vi "TX_单音扫频.vi"() -> ()   [LabVIEW 2015]
uses:
  <vilib>/Instr/_visa.llb/VISA Configure Serial Port (Instr).vi
  <instrlib>/Agilent E363X Series/Agilent E363X Series.lvlib
  <instrlib>/Rohde&Schwarz Spectrum Analyzer/Rohde&Schwarz Spectrum Analyzer.lvlib
panel:
  in  "type specifier VI Refnum (for type only)":refnum<vi>
  in  "Stop Frequency (0.0) 2":dbl=2130000000.0 caption="Stop Frequency (0.0)" format="%#.9p"
  in  "Start Frequency (0.0) 2":dbl=2000000000.0 caption="Start Frequency (0.0)" format="%#.9p"
  in  "Stop Frequency (0.0)":dbl=2130000000.0 format="%#.9p"
  in  "Start Frequency (0.0)":dbl=2000000000.0 format="%#.9p"
  in  "模板路径 2":path=path "E:/Everst_TestReport/Everst_TestReport_Template.xlsx"
  in  "测试板编号 2":i32=4
  in  "保存路径 2":path=path "E:/Everst_TestReport/Report/Everrst_#"
  in  "开关":bool[](array[boolean])=[FALSE, TRUE, TRUE, FALSE, FALSE, FALSE, FALSE, TRUE, TRUE, FALSE]
  out "volt2v":dbl[](array[numeric])
  out "volt1v3":dbl[](array[numeric])
  in  "error in (no error) 6":errorcluster {"code" format="%.0x"}
  in  "error in (no error) 5":errorcluster caption="error in (no error)"
  in  "error in (no error) 4":errorcluster caption="error in (no error)"
  in  "error in (no error) 3":errorcluster
  in  "error in (no error) 2":errorcluster
  in  "error in (no error)":errorcluster
  in  "直流电源2v":refnum<visa-resource-name>="GPIB0::6::INSTR"
  in  "Frequency (1.0e9 Hz)":dbl=10000000.0 format="%.3f"
  in  "RF Output Level (-30.0 dBm)":dbl=10.0 caption="RF Output Level (-30.0)" format="%.3f"
  in  "Reference Level Offset (0.0) 2":dbl=0.95 caption="Reference Level Offset (0.0)" format="%^.3e"
  in  "Coupling Value (0.0) 2":dbl=200000.0 caption="Coupling Value (0.0)" format="%^.3e"
  in  "Reference Level (-20.0) 2":dbl=30.0 caption="Reference Level (-20.0)" format="%^.3e"
  in  "Span (0.0) 2":dbl=1000000000.0 caption="Span (0.0)" format="%.1f"
  in  "Center Frequency (0.0) 2":dbl=2100000000.0 caption="Center Frequency (0.0)" format="%#.9p"
  in  "Reference Level Offset (0.0)":dbl=2.3 format="%^.3e"
  in  "Coupling Value (0.0)":dbl=200000.0 format="%^.3e"
  in  "Reference Level (-20.0)":dbl=30.0 format="%^.3e"
  in  "Span (0.0)":dbl=1000000000.0 format="%.1f"
  in  "Center Frequency (0.0)":dbl=2100000000.0 format="%#.9p"
  in  "配置文件路径":path=path "E:/Everst_TestReport/config.xlsx"
  out "Bamp_next":dbl[](array[numeric])
  out "Bamp_max":dbl[](array[numeric])
  in  "Marker Search 4":i32(ring)=1 caption="Marker Search" items=["Peak Maximum"=1, "Peak Minimum"=2, "Next Maximum"=3, "Left Maximum"=4, "Right Maximum"=5, "Next Minimum"=6, "Left Minimum"=7, "Right Minimum"=8]
  in  "Peak Excursion 4":dbl=3.0 caption="Peak Excursion" format="%.1f"
  out "channelB_y1":dbl[](array[numeric]) caption="Amplitude" format="%^.3e"
  out "channelB_x1":dbl[](array[numeric]) caption="X" format="%^.3e"
  out "Apos_next":dbl[](array[numeric])
  in  "Aamp_next":dbl[](array[numeric])
  out "Aamp_max":dbl[](array[numeric])
  out "Apos_max":dbl[](array[numeric])
  in  "Marker Search 3":i32(ring)=1 caption="Marker Search" items=["Peak Maximum"=1, "Peak Minimum"=2, "Next Maximum"=3, "Left Maximum"=4, "Right Maximum"=5, "Next Minimum"=6, "Left Minimum"=7, "Right Minimum"=8]
  in  "Peak Excursion 3":dbl=3.0 caption="Peak Excursion" format="%.1f"
  out "channelA_y1":dbl[](array[numeric]) caption="Amplitude" format="%^.3e"
  out "channelA_x1":dbl[](array[numeric]) caption="X" format="%^.3e"
  out "fin_dac":dbl[](array[numeric])
  in  "信号发生器地址":refnum<visa-resource-name>="GPIB0::10::INSTR"
  in  "频谱仪地址B":refnum<visa-resource-name>="TCPIP0::192.168.1.4::inst0::INSTR"
  in  "频谱仪地址A":refnum<visa-resource-name>="GPIB0::22::INSTR"
  in  "直流电源(1.3V)":refnum<visa-resource-name>="GPIB0::4::INSTR"
  in  "FPGA串口地址":refnum<visa-resource-name>="COM3"
  out "fin":dbl[](array[numeric])
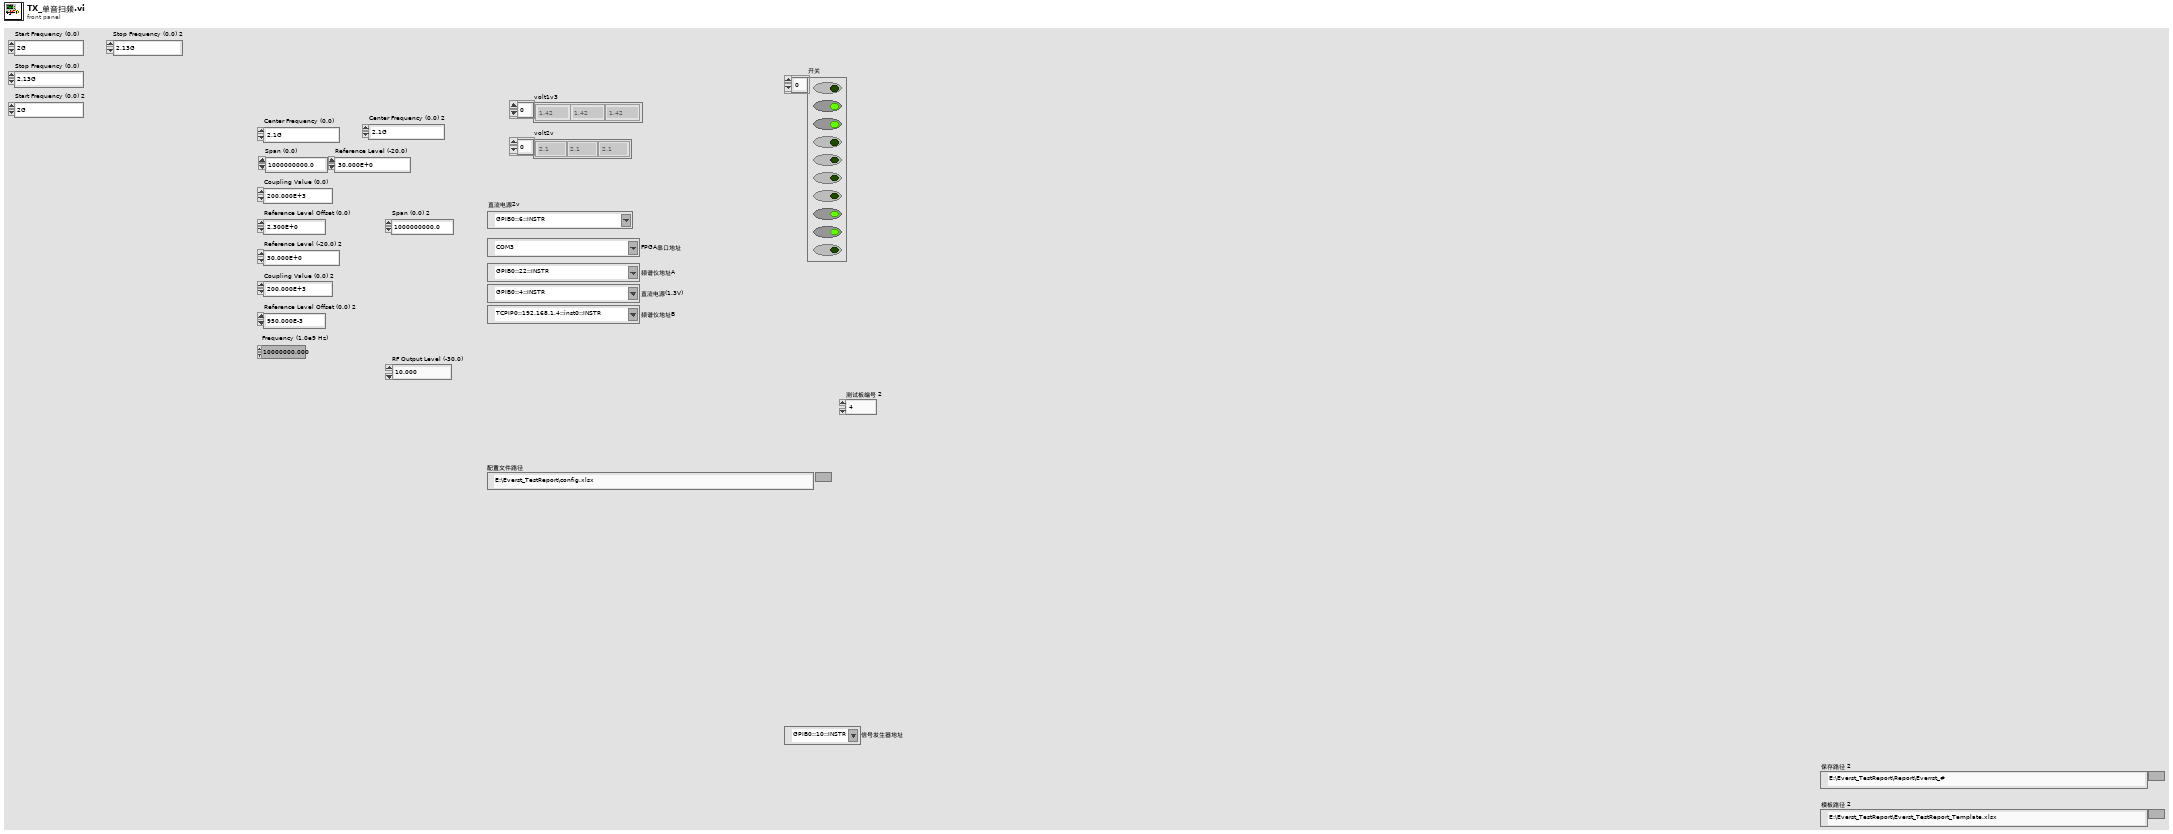
[diagram p1: front panel]
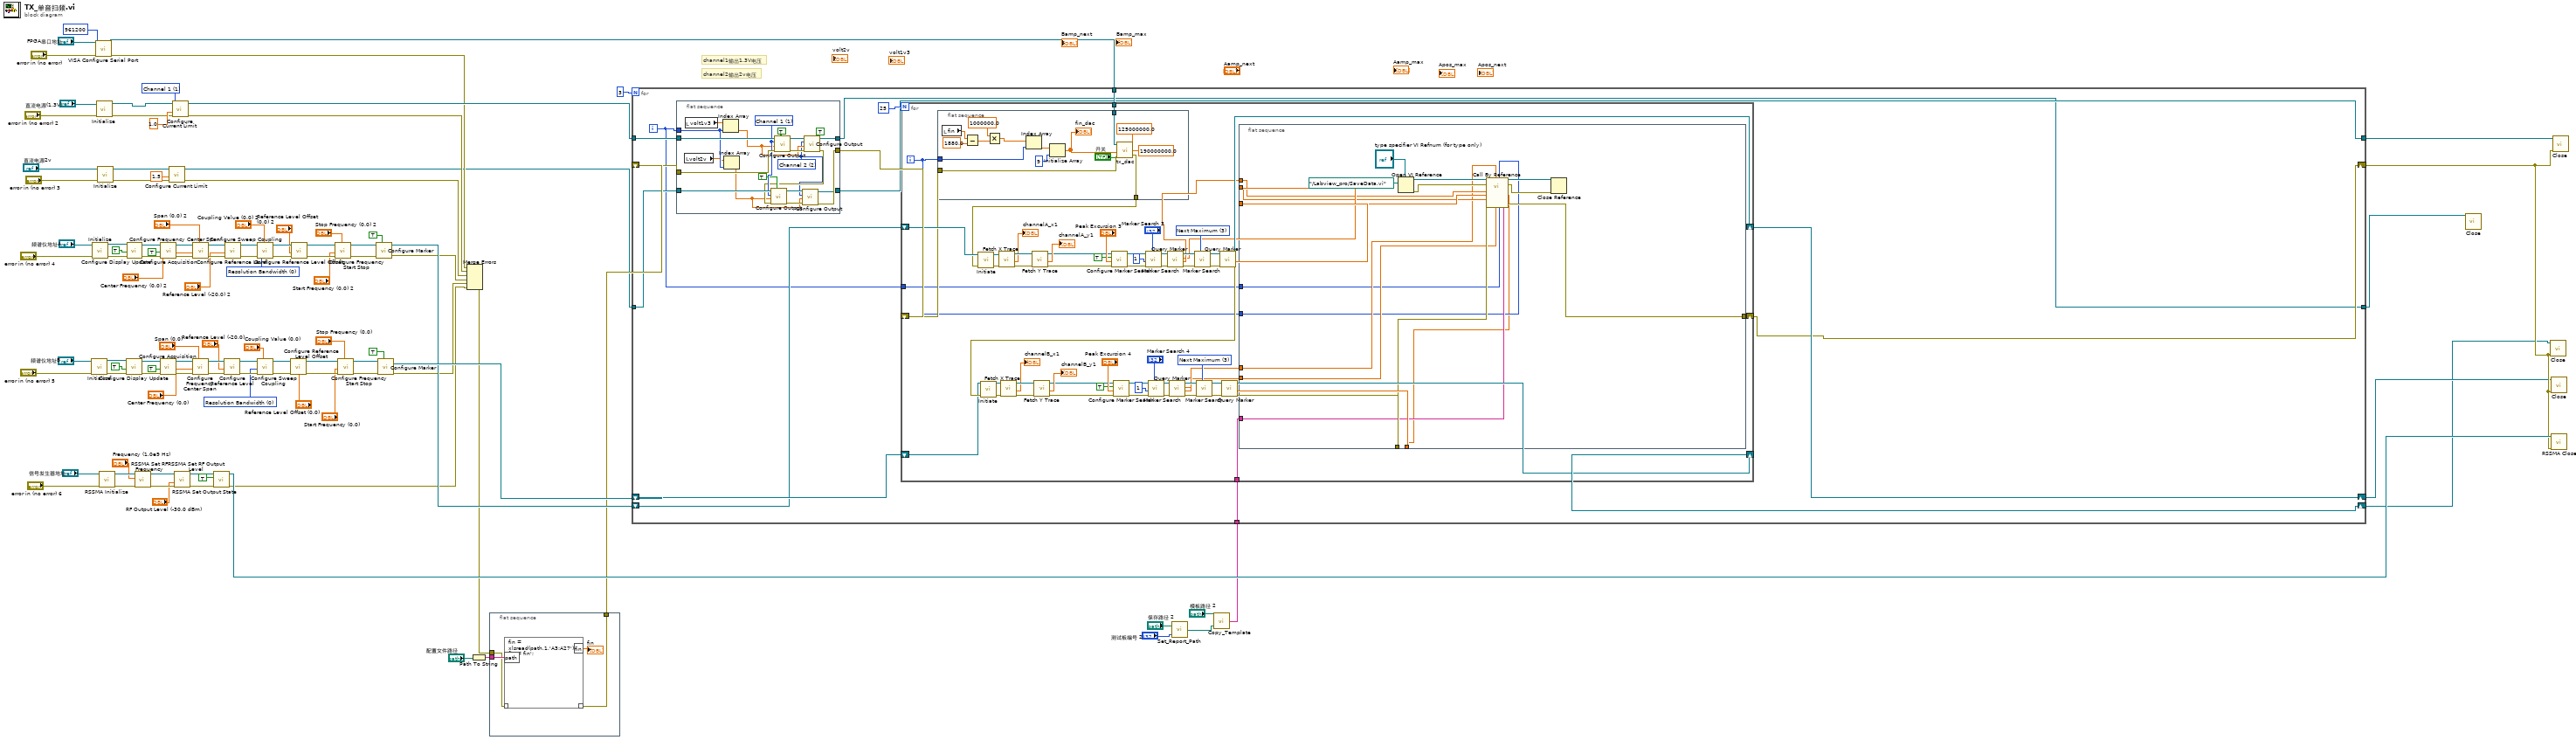
[diagram p0: block diagram]
diagram:
  w39 = 1 items=["Channel 1"=1, "Channel 2"=2, "Channel 3"=3] ("Channel (1: Channel 1)")
  w47 = 0 items=["Resolution Bandwidth", "Video Bandwidth", "Sweep Time"] ("Sweep Coupling (Resolution Bandwidth)")
  w69 = 0 items=["Resolution Bandwidth", "Video Bandwidth", "Sweep Time"] ("Sweep Coupling (Resolution Bandwidth)")
  # "channel2输出2v电压"
  # "channel1输出1.3V电压"
  n1 = call <instrlib>:"Initialize.vi"("VISA resource name"="频谱仪地址B", "error in (no error)"="error in (no error) 5") -> ("VISA resource name out"=w85:refnum<visa-resource-name>, "error out"=w86:errorcluster)  [unwired: 12 in]
  n2 = call <instrlib>:"Initialize.vi"("VISA resource name"="频谱仪地址A", "error in (no error)"="error in (no error) 4") -> ("VISA resource name out"=w63:refnum<visa-resource-name>, "error out"=w64:errorcluster)  [unwired: 12 in]
  n3 = call-poly "VISA Configure Serial Port"("VISA resource name"="FPGA串口地址", "baud rate (9600)"=u32 961200, "error in (no error)"="error in (no error)") -> ("VISA resource name out"=w109:refnum<visa-resource-name>, "error out"=w33:errorcluster)  [unwired: 11 in]
  n4 = call <instrlib>:"Initialize.vi"("error in (no error)"="error in (no error) 2", "VISA resource name"="直流电源(1.3V)") -> ("error out"=w36:errorcluster, "VISA resource name out"=w37:refnum<visa-resource-name>)  [unwired: 8 in]
  n5 = call <instrlib>:"Initialize.vi"("error in (no error)"="error in (no error) 3", "VISA resource name"="直流电源2v") -> ("error out"=w44:errorcluster, "VISA resource name out"=w43:refnum<visa-resource-name>)  [unwired: 8 in]
  n6 = call <instrlib>:"RSSMA Initialize.vi"("error in (no error)"="error in (no error) 6", "Resource Name (GPIB::28)"="信号发生器地址") -> ("error out"=w97:errorcluster, "dup VISA session"=w96:refnum<visa-resource-name>)  [unwired: 8 in]
  n7 = call <instrlib>:"Configure Display Update.vi"("error in (no error)"=w86, "Display In Remote (F: Off)"=TRUE, "VISA resource name"=w85) -> ("error out"=w84:errorcluster, "VISA resource name out"=w83:refnum<visa-resource-name>)  [unwired: 7 in]
  n8 = call <instrlib>:"Configure Display Update.vi"("error in (no error)"=w64, "Display In Remote (F: Off)"=TRUE, "VISA resource name"=w63) -> ("error out"=w62:errorcluster, "VISA resource name out"=w61:refnum<visa-resource-name>)  [unwired: 7 in]
  n9 = call <instrlib>:"RSSMA Set RF Frequency.vi"("error in (no error)"=w97, "Frequency (1.0e9 Hz)"="Frequency (1.0e9 Hz)", "VISA session"=w96) -> ("error out"=w94:errorcluster, "dup VISA session"=w93:refnum<visa-resource-name>)  [unwired: 7 in]
  n10 = call <instrlib>:"Configure Acquisition.vi"("error in (no error)"=w84, "Sweep Mode Continuous (F: Off)"=TRUE, "VISA resource name"=w83) -> ("error out"=w81:errorcluster, "VISA resource name out"=w80:refnum<visa-resource-name>)  [unwired: 7 in]
  n11 = call <instrlib>:"Configure Acquisition.vi"("error in (no error)"=w62, "Sweep Mode Continuous (F: Off)"=TRUE, "VISA resource name"=w61) -> ("error out"=w59:errorcluster, "VISA resource name out"=w58:refnum<visa-resource-name>)  [unwired: 7 in]
  n12 = call <instrlib>:"Configure Current Limit.vi"("error in (no error)"=w44, "Current Limit (0.0 A)"=1.5, "VISA resource name"=w43) -> ("error out"=w31:errorcluster, "VISA resource name out"=w15:refnum<visa-resource-name>)  [unwired: 7 in]
  n13 = call <instrlib>:"Configure Current Limit.vi"("error in (no error)"=w36, "Current Limit (0.0 A)"=1.0, "Channel (1: Channel 1)"=w39, "VISA resource name"=w37) -> ("error out"=w32:errorcluster, "VISA resource name out"=w110:refnum<visa-resource-name>)  [unwired: 6 in]
  n14 = call <instrlib>:"RSSMA Set RF Output Level.vi"("error in (no error)"=w94, "RF Output Level (-30.0 dBm)"="RF Output Level (-30.0 dBm)", "VISA session"=w93) -> ("error out"=w92:errorcluster, "dup VISA session"=w91:refnum<visa-resource-name>)  [unwired: 7 in]
  n15 = call <instrlib>:"Configure Frequency Center Span.vi"("Span (0.0)"="Span (0.0)", "error in (no error)"=w81, "Center Frequency (0.0)"="Center Frequency (0.0)", "VISA resource name"=w80) -> ("error out"=w79:errorcluster, "VISA resource name out"=w78:refnum<visa-resource-name>)  [unwired: 6 in]
  n16 = call <instrlib>:"Configure Frequency Center Span.vi"("Span (0.0)"="Span (0.0) 2", "error in (no error)"=w59, "Center Frequency (0.0)"="Center Frequency (0.0) 2", "VISA resource name"=w58) -> ("error out"=w57:errorcluster, "VISA resource name out"=w56:refnum<visa-resource-name>)  [unwired: 6 in]
  n17 = call <instrlib>:"RSSMA Set Output State.vi"("error in (no error)"=w92, "RF Output State (F: Off)"=TRUE, "VISA session"=w91) -> ("error out"=w28:errorcluster, "dup VISA session"=w108:refnum<visa-resource-name>)  [unwired: 7 in]
  n18 = call <instrlib>:"Configure Reference Level.vi"("error in (no error)"=w79, "Reference Level (-20.0)"="Reference Level (-20.0)", "VISA resource name"=w78) -> ("error out"=w77:errorcluster, "VISA resource name out"=w76:refnum<visa-resource-name>)  [unwired: 7 in]
  n19 = call <instrlib>:"Configure Reference Level.vi"("error in (no error)"=w57, "Reference Level (-20.0)"="Reference Level (-20.0) 2", "VISA resource name"=w56) -> ("error out"=w55:errorcluster, "VISA resource name out"=w54:refnum<visa-resource-name>)  [unwired: 7 in]
  n20 = call <instrlib>:"Configure Sweep Coupling.vi"("Coupling Value (0.0)"="Coupling Value (0.0)", "error in (no error)"=w77, "Sweep Coupling (Resolution Bandwidth)"=w69, "VISA resource name"=w76) -> ("error out"=w75:errorcluster, "VISA resource name out"=w74:refnum<visa-resource-name>)  [unwired: 6 in]
  n21 = call <instrlib>:"Configure Sweep Coupling.vi"("Coupling Value (0.0)"="Coupling Value (0.0) 2", "error in (no error)"=w55, "Sweep Coupling (Resolution Bandwidth)"=w47, "VISA resource name"=w54) -> ("error out"=w53:errorcluster, "VISA resource name out"=w52:refnum<visa-resource-name>)  [unwired: 6 in]
  n22 = call <instrlib>:"Configure Reference Level Offset.vi"("error in (no error)"=w75, "Reference Level Offset (0.0)"="Reference Level Offset (0.0)", "VISA resource name"=w74) -> ("error out"=w9:errorcluster, "VISA resource name out"=w8:refnum<visa-resource-name>)  [unwired: 7 in]
  n23 = call <instrlib>:"Configure Reference Level Offset.vi"("error in (no error)"=w53, "Reference Level Offset (0.0)"="Reference Level Offset (0.0) 2", "VISA resource name"=w52) -> ("error out"=w13:errorcluster, "VISA resource name out"=w12:refnum<visa-resource-name>)  [unwired: 7 in]
  n24 = call <instrlib>:"Configure Frequency Start Stop.vi"("Stop Frequency (0.0)"="Stop Frequency (0.0) 2", "error in (no error)"=w13, "Start Frequency (0.0)"="Start Frequency (0.0) 2", "VISA resource name"=w12) -> ("error out"=w11:errorcluster, "VISA resource name out"=w10:refnum<visa-resource-name>)  [unwired: 6 in]
  n25 = call <instrlib>:"Configure Frequency Start Stop.vi"("Stop Frequency (0.0)"="Stop Frequency (0.0)", "error in (no error)"=w9, "Start Frequency (0.0)"="Start Frequency (0.0)", "VISA resource name"=w8) -> ("error out"=w7:errorcluster, "VISA resource name out"=w6:refnum<visa-resource-name>)  [unwired: 6 in]
  n26 = call <instrlib>:"Configure Marker.vi"("Marker State (F: Off)"=TRUE, "error in (no error)"=w11, "VISA resource name"=w10) -> ("error out"=w30:errorcluster, "VISA resource name out"=w103:refnum<visa-resource-name>)  [unwired: 7 in]
  n27 = call <instrlib>:"Configure Marker.vi"("Marker State (F: Off)"=TRUE, "error in (no error)"=w7, "VISA resource name"=w6) -> ("error out"=w29:errorcluster, "VISA resource name out"=w104:refnum<visa-resource-name>)  [unwired: 7 in]
  n28 = Merge Errors(w33, w32, w31, w30, w29, w28) -> (w21:errorcluster)
  n29 = Path To String(path="配置文件路径") -> (string=w100:string)
  n30 = flat-sequence {
    tunnel: w100 -> [w113]
    tunnel: w21 -> [w112]
    tunnel: [w111] -> w20
    frame #0 {
      n31 = script code="fin = xlsread(path,1,'A3:A27');\nfin = fin';"("??"=w112, "path"=w113) -> ("??"=w111:errorcluster, "fin"=→"fin":dbl[])
    }
  }
  n32 = call "Set_Report_Path.vi"("测试板编号"="测试板编号 2", "保存路径"="保存路径 2") -> ("创建生成路径"=w18:path)
  n33 = call "Copy_Template.vi"("报告保存路径"=w18, "模板路径"="模板路径 2") -> ("报告保存路径字符串"=w14:string)
  n34 = for {
    N: 3 -> [_]
    tunnel: w109 -> [w128]
    shift-right: [w120] -> w106
    shift-left: w20 -> [w127]
    shift-right: [w126] -> w105
    shift-left: w104 -> [w125]
    shift-right: [w123] -> w102
    shift-left: w103 -> [w124]
    tunnel: w14 -> [w116]
    tunnel: w110 -> [w129]
    tunnel: [w119] -> w107
    tunnel: w15 -> [w117]
    tunnel: [w118] -> w16
    i -> [w115]
    n35 = flat-sequence {
      tunnel: w129 -> [w242]
      tunnel: w127 -> [w240]
      tunnel: w117 -> [w239]
      tunnel: [w231] -> w121
      tunnel: [w235] -> w118
      tunnel: [w227] -> w119
      tunnel: w115 -> [w225]
      frame #0 {
        w226 = 2 items=["Channel 1"=1, "Channel 2"=2, "Channel 3"=3] ("Channel (1: Channel 1)")
        (unwired) TRUE ("Enable Output (T: Enable)")
        w238 = 1 items=["Channel 1"=1, "Channel 2"=2, "Channel 3"=3] ("Channel (1: Channel 1)")
        n36 = local read "volt2v"() -> (w223:dbl[])
        n37 = local read "volt1v3"() -> (w224:dbl[])
        n38 = Index Array(array=w224, index=w225) -> (element=w230:dbl)
        n39 = Index Array(array=w223, index=w225) -> (element=w229:dbl)
        n40 = call <instrlib>:"Configure Output.vi"("Enable Output (T: Enable)"=TRUE, "error in (no error)"=w240, "Voltage Level (0.0 V)"=w230, "Channel (1: Channel 1)"=w238, "VISA resource name"=w242) -> ("error out"=w234:errorcluster, "VISA resource name out"=w236:refnum<visa-resource-name>)  [unwired: 5 in]
        n41 = call <instrlib>:"Configure Output.vi"("error in (no error)"=w234, "Voltage Level (0.0 V)"=w230, "Channel (1: Channel 1)"=w226, "VISA resource name"=w236) -> ("error out"=w233:errorcluster, "VISA resource name out"=w235:refnum<visa-resource-name>)  [unwired: 6 in]
        n42 = call <instrlib>:"Configure Output.vi"("Enable Output (T: Enable)"=TRUE, "error in (no error)"=w233, "Voltage Level (0.0 V)"=w229, "Channel (1: Channel 1)"=w238, "VISA resource name"=w239) -> ("error out"=w232:errorcluster, "VISA resource name out"=w228:refnum<visa-resource-name>)  [unwired: 5 in]
        n43 = call <instrlib>:"Configure Output.vi"("error in (no error)"=w232, "Voltage Level (0.0 V)"=w229, "Channel (1: Channel 1)"=w226, "VISA resource name"=w228) -> ("error out"=w231:errorcluster, "VISA resource name out"=w227:refnum<visa-resource-name>)  [unwired: 6 in]
      }
    }
    n44 = for {
      N: 25 -> [_]
      tunnel: w128 -> [w190]
      shift-right: [w130] -> w120
      shift-left: w121 -> [w186]
      shift-right: [w185] -> w126
      shift-left: w124 -> [w189]
      shift-right: [w183] -> w123
      shift-left: w125 -> [w184]
      tunnel: w116 -> [w135]
      tunnel: w115 -> [w133]
      i -> [w134]
      w141 = 3 items=["Peak Maximum"=1, "Peak Minimum"=2, "Next Maximum"=3, "Left Maximum"=4, "Right Maximum"=5, "Next Minimum"=6, "Left Minimum"=7, "Right Minimum"=8] ("Marker Search (Peak Maximum)")
      w162 = 3 items=["Peak Maximum"=1, "Peak Minimum"=2, "Next Maximum"=3, "Left Maximum"=4, "Right Maximum"=5, "Next Minimum"=6, "Left Minimum"=7, "Right Minimum"=8] ("Marker Search (Peak Maximum)")
      n45 = flat-sequence {
        tunnel: w134 -> [w220]
        tunnel: w190 -> [w219]
        tunnel: w186 -> [w216]
        tunnel: [w215] -> w188
        frame #0 {
          n46 = local read "fin"() -> (w222:dbl[])
          n47 = Subtract(x=w222, y=1880.0) -> (x-y=w213:dbl[])
          n48 = Multiply(x=1000000.0, y=w213) -> (x*y=w212:dbl[])
          n49 = Index Array(array=w212, index=w220) -> (element=w209:dbl)
          n50 = Initialize Array(w209, 9 ("dimension size")) -> (w208:dbl[])
          "fin_dac" <- w208
          n51 = call "tx_dac.vi"("fnco"=190000000.0, "fs"=125000000.0, "error in (no error)"=w216, "fin"=w208, "开关"="开关", "VISA resource name 2"=w219) -> ("error out"=w215:errorcluster)
        }
      }
      n52 = call <instrlib>:"Initiate.vi"("error in (no error)"=w188, "VISA resource name"=w189) -> ("error out"=w167:errorcluster, "VISA resource name out"=w168:refnum<visa-resource-name>)  [unwired: 8 in]
      n53 = call <instrlib>:"Fetch X Trace.vi"("error in (no error)"=w167, "VISA resource name"=w168) -> ("error out"=w181:errorcluster, "X"=→"channelA_x1":dbl[], "VISA resource name out"=w182:refnum<visa-resource-name>)  [unwired: 7 in]
      n54 = call <instrlib>:"Fetch Y Trace.vi"("error in (no error)"=w181, "VISA resource name"=w182) -> ("error out"=w169:errorcluster, "Amplitude"=→"channelA_y1":dbl[], "VISA resource name out"=w170:refnum<visa-resource-name>)  [unwired: 7 in]
      n55 = call <instrlib>:"Configure Marker Search.vi"("error in (no error)"=w169, "Peak Excursion (6.0)"="Peak Excursion 3", "Local Oscillator Supression (T: On)"=TRUE ("Local Oscillator Supression (On)"), "VISA resource name"=w170) -> ("error out"=w175:errorcluster, "VISA resource name out"=w174:refnum<visa-resource-name>)  [unwired: 6 in]
      n56 = call <instrlib>:"Marker Search.vi"("Marker Search (Peak Maximum)"="Marker Search 3", "error in (no error)"=w175, "Marker (1)"=1, "VISA resource name"=w174) -> ("error out"=w172:errorcluster, "VISA resource name out"=w173:refnum<visa-resource-name>)  [unwired: 6 in]
      n57 = call <instrlib>:"Query Marker.vi"("error in (no error)"=w172, "VISA resource name"=w173) -> ("error out"=w166:errorcluster, "Marker Amplitude"=w140:dbl, "Marker Position"=w132:dbl, "VISA resource name out"=w165:refnum<visa-resource-name>)  [unwired: 6 in]
      n58 = call <instrlib>:"Marker Search.vi"("Marker Search (Peak Maximum)"=w162, "error in (no error)"=w166, "VISA resource name"=w165) -> ("error out"=w164:errorcluster, "VISA resource name out"=w163:refnum<visa-resource-name>)  [unwired: 7 in]
      n59 = call <instrlib>:"Query Marker.vi"("error in (no error)"=w164, "VISA resource name"=w163) -> ("error out"=w187:errorcluster, "Marker Amplitude"=w139:dbl, "VISA resource name out"=w185:refnum<visa-resource-name>)  [unwired: 6 in, 1 out]
      n60 = call <instrlib>:"Initiate.vi"("error in (no error)"=w187, "VISA resource name"=w184) -> ("error out"=w146:errorcluster, "VISA resource name out"=w147:refnum<visa-resource-name>)  [unwired: 8 in]
      n61 = call <instrlib>:"Fetch X Trace.vi"("error in (no error)"=w146, "VISA resource name"=w147) -> ("error out"=w160:errorcluster, "X"=→"channelB_x1":dbl[], "VISA resource name out"=w161:refnum<visa-resource-name>)  [unwired: 7 in]
      n62 = call <instrlib>:"Fetch Y Trace.vi"("error in (no error)"=w160, "VISA resource name"=w161) -> ("error out"=w148:errorcluster, "Amplitude"=→"channelB_y1":dbl[], "VISA resource name out"=w149:refnum<visa-resource-name>)  [unwired: 7 in]
      n63 = call <instrlib>:"Configure Marker Search.vi"("error in (no error)"=w148, "Peak Excursion (6.0)"="Peak Excursion 4", "Local Oscillator Supression (T: On)"=TRUE ("Local Oscillator Supression (On)"), "VISA resource name"=w149) -> ("error out"=w154:errorcluster, "VISA resource name out"=w153:refnum<visa-resource-name>)  [unwired: 6 in]
      n64 = call <instrlib>:"Marker Search.vi"("Marker Search (Peak Maximum)"="Marker Search 4", "error in (no error)"=w154, "Marker (1)"=1, "VISA resource name"=w153) -> ("error out"=w151:errorcluster, "VISA resource name out"=w152:refnum<visa-resource-name>)  [unwired: 6 in]
      n65 = call <instrlib>:"Query Marker.vi"("error in (no error)"=w151, "VISA resource name"=w152) -> ("error out"=w145:errorcluster, "Marker Amplitude"=w138:dbl, "Marker Position"=w131:dbl, "VISA resource name out"=w144:refnum<visa-resource-name>)  [unwired: 6 in]
      n66 = call <instrlib>:"Marker Search.vi"("Marker Search (Peak Maximum)"=w141, "error in (no error)"=w145, "VISA resource name"=w144) -> ("error out"=w143:errorcluster, "VISA resource name out"=w142:refnum<visa-resource-name>)  [unwired: 7 in]
      n67 = call <instrlib>:"Query Marker.vi"("error in (no error)"=w143, "VISA resource name"=w142) -> ("error out"=w136:errorcluster, "Marker Amplitude"=w137:dbl, "VISA resource name out"=w183:refnum<visa-resource-name>)  [unwired: 6 in, 1 out]
      n68 = flat-sequence {
        tunnel: w140 -> [w201]
        tunnel: w139 -> [w200]
        tunnel: w138 -> [w195]
        tunnel: w137 -> [w191]
        tunnel: w136 -> [w198]
        tunnel: w135 -> [w196]
        tunnel: w134 -> [w193]
        tunnel: w133 -> [w192]
        tunnel: w132 -> [w199]
        tunnel: w131 -> [w194]
        tunnel: [w197] -> w130
        frame #0 {
          n69 = Open VI Reference(type specifier VI Refnum (for type only)="type specifier VI Refnum (for type only)", vi path=path "../Labview_pro/SaveData.vi") -> (vi reference=w206:refnum<vi>, error out=w205:errorcluster)  [unwired: 4 in]
          n70 = call-by-ref "?"(reference=w206, error in=w205, "Bamp_next"=w191, "path"=w196, "index"=w192, "Findex"=w193, "Bmax_pos"=w194, "Bamp_max"=w195, "error in"=w198, "Amax_pos"=w199, "Aamp_next"=w200, "Aamp_max"=w201) -> (reference out=w202:refnum<vi>, error out=w203:errorcluster, 0:"error out"=w197:errorcluster)  [unwired: 1 in]
          n71 = Close Reference(reference=w202, error in (no error)=w203) -> ()  [unwired: 1 out]
        }
      }
    }
  }
  n72 = call <instrlib>:"Close.vi"("VISA resource name"=w16) -> ()  [unwired: 10 in, 1 out]
  n73 = call <instrlib>:"Close.vi"("error in (no error)"=w106, "VISA resource name"=w102) -> ()  [unwired: 9 in, 1 out]
  n74 = call <instrlib>:"Close.vi"("error in (no error)"=w106, "VISA resource name"=w105) -> ()  [unwired: 9 in, 1 out]
  n75 = call <instrlib>:"RSSMA Close.vi"("error in (no error)"=w106, "VISA session"=w108) -> ()  [unwired: 9 in, 1 out]
  n76 = call <instrlib>:"Close.vi"("error in (no error)"=w106, "VISA resource name"=w107) -> ()  [unwired: 9 in, 1 out]
